vi "FilterLidar.vi"(9 "WhatAroundMeMap? Last 2":cluster{"T":dbl, "Range":dbl, "Bearing":dbl}[](array[cluster]), 10 "WhatAroundMeMap? Last 3":cluster{"T":dbl, "Range":dbl, "Bearing":dbl}[](array[cluster]), 11 "WhatAroundMeMap? Last":cluster{"T":dbl, "Range":dbl, "Bearing":dbl}[](array[cluster])) -> (3 "WhatAroundMeMap?":cluster{"T":dbl, "Range":dbl, "Bearing":dbl}[](array[cluster]))   [LabVIEW 2012]
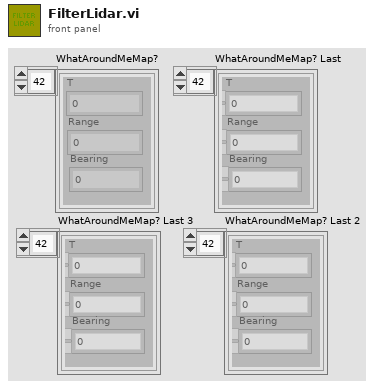
[diagram p1: front panel]
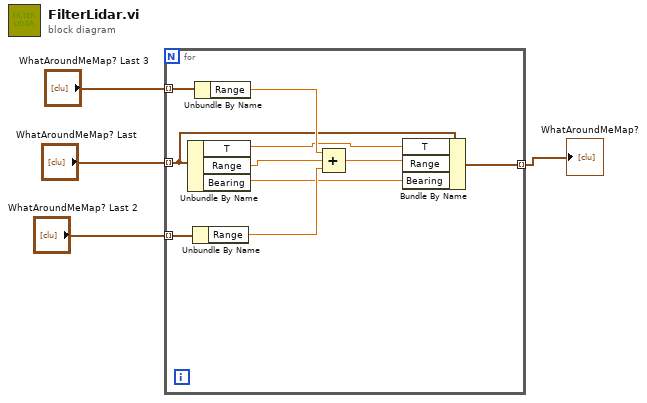
[diagram p0: block diagram]
diagram:
  n1 = for {
    tunnel: "WhatAroundMeMap? Last 3" -> [w13] mode=indexing
    tunnel: "WhatAroundMeMap? Last" -> [w8] mode=indexing
    tunnel: "WhatAroundMeMap? Last 2" -> [w14] mode=indexing
    tunnel: [w5] -> w1 mode=indexing
    n2 = Unbundle By Name(w8) -> ("T"=w7:dbl, "Range"=w10:dbl, "Bearing"=w6:dbl)
    n3 = Unbundle By Name(w14) -> ("Range"=w12:dbl)
    n4 = Unbundle By Name(w13) -> ("Range"=w11:dbl)
    n5 = Compound Arithmetic op=ADD(w11, w10, w12) -> (w9:dbl)
    n6 = Bundle By Name(cluster=w8, "T"=w7, "Range"=w9, "Bearing"=w6) -> (w5:cluster{"T":dbl, "Range":dbl, "Bearing":dbl})
  }
  "WhatAroundMeMap?" <- w1
